vi "Get Next Data.vi"(8 "error in (no error)":errorcluster, 11 "Data Plugin in":refnum<class "Data Plugin.lvclass">) -> (0 "error out":errorcluster, 2 "Data":dbl, 3 "Data Plugin out":refnum<class "Data Plugin.lvclass">)   [LabVIEW 2017, in "Data Engine.lvlib" / "Data Plugin.lvclass"]
uses:
  Data Plugin.lvclass
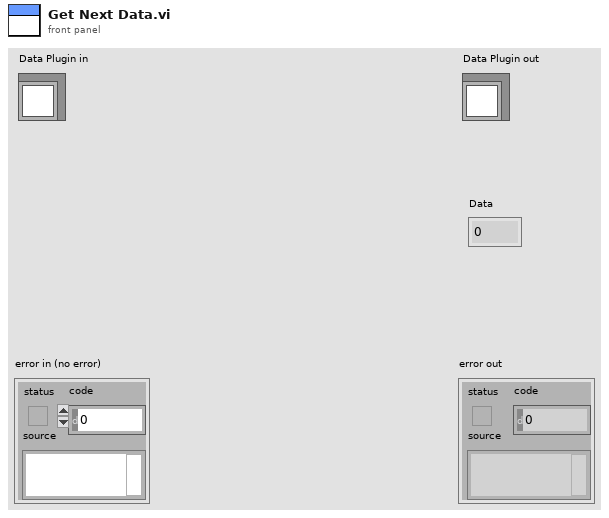
[diagram p1: front panel]
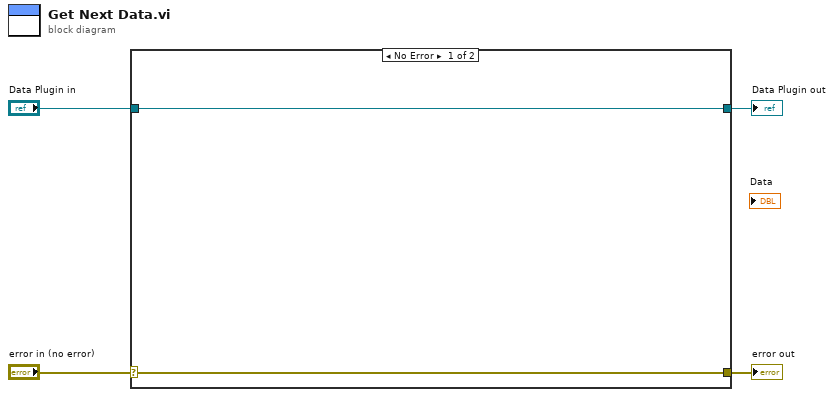
[diagram p0: block diagram]
diagram:
  n1 = case shown="No Error" "error in (no error)" {
    selector: "error in (no error)" -> [w5 w8]
    tunnel: [w5 w8] -> w3
    tunnel: [w6 w7] -> w1
    tunnel: "Data Plugin in" -> [w6 w7]
    frame No Error {
    }
    frame Error {
    }
  }
  "error out" <- w3
  "Data Plugin out" <- w1
